vi "test_generic.vi"() -> (0 "error out":errorcluster)   [LabVIEW 2010, in "GenericInstrument.lvclass"]
uses:
  GenericInstrument.lvclass
  main/labview_source/type_definitions/clusters/controls_refs.ctl
  common/classes/ErrorController/ErrorController/ErrorController.lvclass
  common/classes/GenericToplevelComponent/GenericToplevelComponent/common_trigger_enum.ctl
  common/classes/XMLElement/XMLElement/XMLElement.lvclass
  common/classes/ErrorController/ErrorController/class_data.vi
  common/classes/GenericComponent/GenericComponent/GenericComponent.lvclass
  common/classes/GenericToplevelComponent/GenericToplevelComponent/GenericToplevelComponent.lvclass
panel:
  out "error loaded?":bool
  in  "create OME XML button":bool
  out "OME XML":string
  in  "scan start button":bool
  in  "create button":bool
  in  "stop button":bool
  # "Test Instrument"
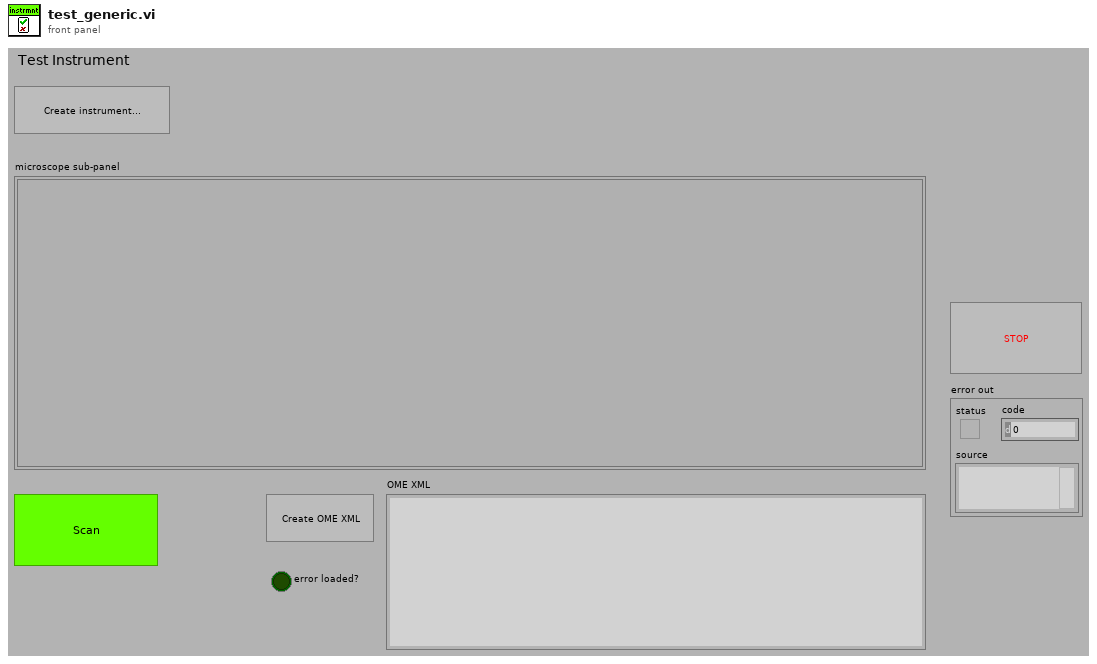
[diagram p1: front panel]
types:
  T1 = typedef "controls_refs.ctl" = cluster{"scan start button":refnum<vi>, "tabs":cluster{"main":refnum<vi>, "settings":refnum<vi>}, "subpanels":cluster{"imagingMode":refnum<vi>, "scanHead":refnum<vi>, "display":refnum<vi>, "experimentController":refnum<vi>, "instrument":refnum<vi>, "stage":refnum<vi>, "stimulator":refnum<vi>, "dataCollection":refnum<vi>, "analyser":refnum<vi>, "daq":refnum<vi>, "imageAssembler":refnum<vi>}, "drop-downs":cluster{"run mode":refnum<vi>, "imagingMode":refnum<vi>, "experimentalController":refnum<vi>, "objective":refnum<vi>}, "status lights":cluster{"experimentController":refnum<vi>, "imagingMode":refnum<vi>, "scanHead":refnum<vi>, "daq":refnum<vi>, "imageAssembler":refnum<vi>, "dataCollection":refnum<vi>, "display":refnum<vi>, "analyser":refnum<vi>, "stage":refnum<vi>, "stimulator":refnum<vi>, "instrument":refnum<vi>}, "message":refnum<vi>, "stimulator enabled?":refnum<vi>, "saving":cluster{"data folder path":refnum<vi>, "file base name":refnum<vi>, "notebook":refnum<vi>}, "progress bar":refnum<vi>, "update icon":refnum<vi>, "title":refnum<vi>, "main vi":refnum<vi>, "user":refnum<vi>, "exit_button":refnum<vi>, "CPU usage %":refnum<vi>}
  T2 = typedef "GenericToplevelComponent.lvclass/common_trigger_enum.ctl" = enum16{"NULL", "initialise", "terminate", "fetch command", "fetch data", "attach observer", "register as observer", "detach observer", "acknowledge", "start", "stop", "sweep started", "sweep finished", "experiment started", "experiment stopped"}
  T3 = typedef "XComponentSpecification.xctl/data.ctl" = cluster{"class path":string, "configuration":string, "label":string, "settings name":string}
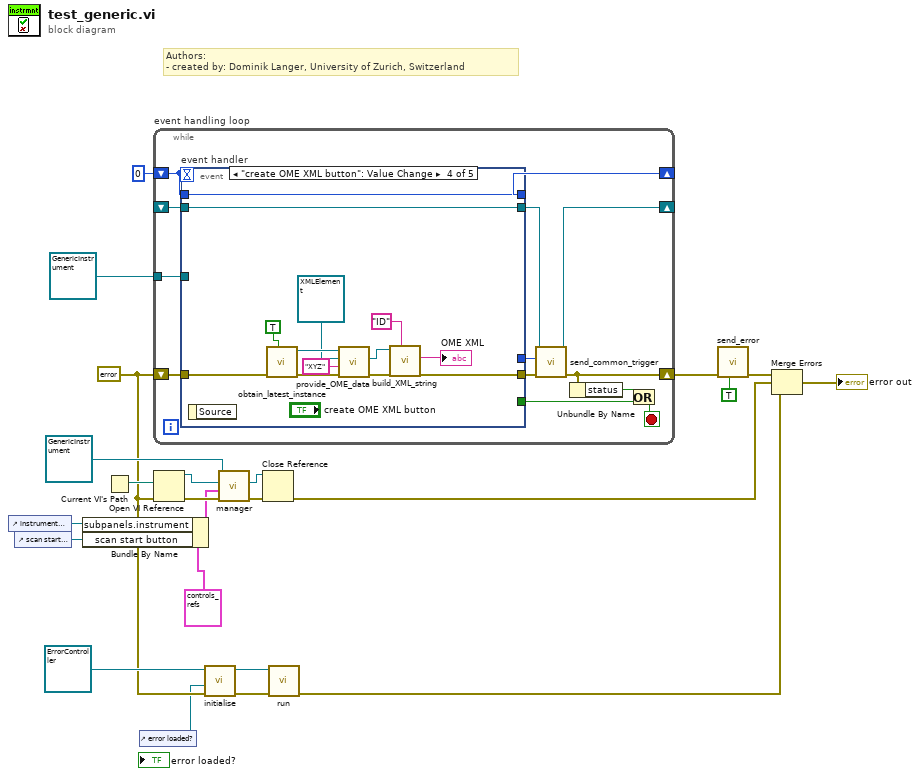
[diagram p0: block diagram]
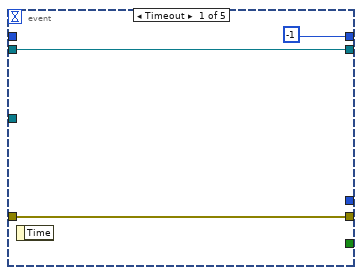
[diagram p2: hidden frame]
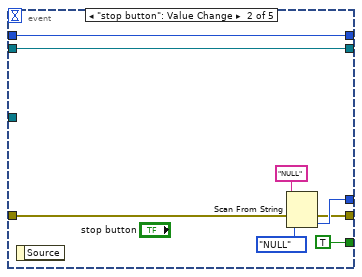
[diagram p3: hidden frame]
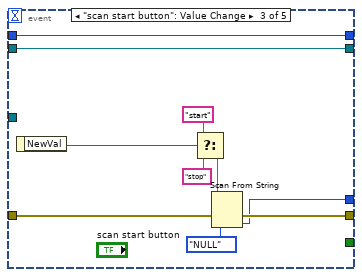
[diagram p4: hidden frame]
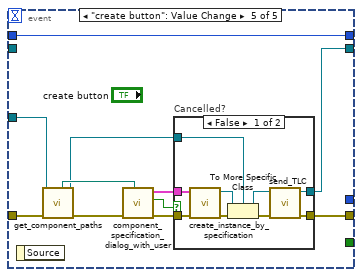
[diagram p5: hidden frame]
diagram:
  w3 = errorcluster {"status"=FALSE, "code"=0, "source"=""} ("error out")
  # "Authors: \n- created by: Dominik Langer, University of Zurich, Switzerland"
  n1 = control-ref of="instrument sub-panel"() -> (w21:refnum<vi>)
  n2 = control-ref of="scan start button"() -> (w19:refnum<vi>)
  n3 = Bundle By Name(cluster=T1 {"scan start button"=refnum, "tabs"={"main"=refnum, "settings"=refnum}, "subpanels"={"imagingMode"=refnum, "scanHead"=refnum, "display"=refnum, "experimentController"=refnum, "instrument"=refnum, "stage"=refnum, "stimulator"=refnum, "dataCollection"=refnum, "analyser"=refnum, "daq"=refnum, "imageAssembler"=refnum}, "drop-downs"={"run mode"=refnum, "imagingMode"=refnum, "experimentalController"=refnum, "objective"=refnum}, "status lights"={"experimentController"=refnum, "imagingMode"=refnum, "scanHead"=refnum, "daq"=refnum, "imageAssembler"=refnum, "dataCollection"=refnum, "display"=refnum, "analyser"=refnum, "stage"=refnum, "stimulator"=refnum, "instrument"=refnum}, "message"=refnum, "stimulator enabled?"=refnum, "saving"={"data folder path"=refnum, "file base name"=refnum, "notebook"=refnum}, "progress bar"=refnum, "update icon"=refnum, "title"=refnum, "main vi"=refnum, "user"=refnum, "exit_button"=refnum, "CPU usage %"=refnum} ("control references"), "subpanels.instrument"=w21, "scan start button"=w19) -> (w14:T1)
  n4 = Current VI's Path() -> (path=w16:path)
  n5 = control-ref of="error loaded?"() -> (w2:refnum<vi>)
  n6 = while "event handling loop" {
    shift-right: [w27] -> w6
    shift-left: w3 -> [w36]
    shift-right: [w34] -> _
    shift-left: 0 -> [w35]
    shift-right: [w30] -> _
    shift-left: _ -> [w33]
    tunnel: refnum<class "GenericInstrument.lvclass"> refnum ("GenericInstrument.lvclass") -> [w28]
    stop <- w25 stop-if-true
    n7 = event "event handler" shown="[3] \"create OME XML button\": Value Change" {
      selector: _ -> [_ _ _ _ _]
      dyn-events: _ -> [_ _ _ _ _]
      timeout: w35 -> [_ _ _ _ _]
      tunnel: w36 -> [w37 w41 w53 w68 w75]
      tunnel: [-1 w47 w57 w70 w81] -> w34
      tunnel: w35 -> [_ w47 w57 w70 w81]
      tunnel: [w37 w40 w52 w61 w80] -> w31
      tunnel: [_ TRUE _ _ _] -> w24
      tunnel: w33 -> [w38 w45 w55 w69 _]
      tunnel: [w38 w45 w55 w69 w79] -> w32
      tunnel: [_ w42 w48 _ _] -> w29
      tunnel: w28 -> [_ _ _ _ w74]
      event Timeout {
        n8 = event-data() -> ()  [unwired: 2 out]
      }
      event "stop button": Value Change {
        n9 = event-data() -> ()  [unwired: 2 out]
        n10 = Scan From String(input string="NULL", error in=w41, default 1=common_trigger_enum."NULL" ("f")) -> (error out=w40:errorcluster, output 1=w42:T2)  [unwired: 2 in, 2 out]
      }
      event "scan start button": Value Change {
        n11 = event-data() -> ("NewVal"=w56:bool)  [unwired: 1 out]
        n12 = Select(t="start", s=w56, f="stop") -> (s? t:f=w51:string)
        n13 = Scan From String(input string=w51, error in=w53, default 1=common_trigger_enum."NULL" ("f")) -> (error out=w52:errorcluster, output 1=w48:T2)  [unwired: 2 in, 2 out]
      }
      event "create OME XML button": Value Change {
        n14 = event-data() -> ()  [unwired: 2 out]
        n15 = call "obtain_latest_instance.vi"("quick, but maybe outdated?"=TRUE, "error in (no error)"=w68) -> ("error out"=w66:errorcluster, "microscope"=w65:refnum<class "GenericInstrument.lvclass">)  [unwired: 8 in]
        n16 = call-dynamic "provide_OME_data.vi"("error in (no error)"=w66, "structuredAttribute string in"="XYZ" ("image ID"), "OME element in"=refnum<class "XMLElement.lvclass"> refnum ("XMLElement.lvclass"), "GenericPlugin in"=w65) -> ("error out"=w62:errorcluster, "OME element out"=w60:refnum<class "XMLElement.lvclass">)  [unwired: 4 in, 2 out]
        n17 = call "build_XML_string.vi"("ID tag"="ID" ("id parameter name"), "error in (no error)"=w62, "Element in"=w60) -> ("error out"=w61:errorcluster, "string"=→"OME XML":string)  [unwired: 6 in, 1 out]
      }
      event "create button": Value Change {
        n18 = event-data() -> ()  [unwired: 2 out]
        n19 = call-dynamic "get_component_paths.vi"("error in (no error)"=w75, "GenericComponent in"=w74) -> ("error out"=w77:errorcluster, "GenericComponent out"=w73:refnum<class "GenericInstrument.lvclass">, "component type directory"=w78:path)  [unwired: 4 in, 3 out]
        n20 = call "component_specification_dialog_with_user.vi"("start path"=w78, "error in (no error)"=w77) -> ("error out"=w76:errorcluster, "cancelled?"=w71:bool, "component specification out"=w72:T3)  [unwired: 7 in]
        n21 = case "Cancelled?" shown="False" w71 {
          tunnel: [w88 w92] -> w80
          tunnel: [w85 w91] -> w79
          tunnel: w76 -> [w84 w92]
          tunnel: w73 -> [w83 w91]
          tunnel: w72 -> [w82 _]
          frame False {
            n22 = call "create_instance_by_specification.vi"("error in (no error)"=w84, "component specification"=w82) -> ("error out"=w90:errorcluster, "GenericPlugin out"=w87:refnum<class "GenericComponent.lvclass">)  [unwired: 7 in, 1 out]
            n23 = To More Specific Class(target class=w83, reference=w87, error in=w90) -> (specific class reference=w86:refnum<class "GenericInstrument.lvclass">, error out=w89:errorcluster)
            n24 = call-dynamic "send_TLC.vi"("error in (no error)"=w89, "GenericToplevelComponent in"=w86) -> ("error out"=w88:errorcluster, "GenericToplevelComponent out"=w85:refnum<class "GenericInstrument.lvclass">)  [unwired: 8 in]
          }
          frame True {
          }
        }
      }
    }
    n25 = call-dynamic "send_common_trigger.vi"("error in (no error)"=w31, "trigger"=w29, "GenericToplevelComponent in"=w32) -> ("error out"=w27:errorcluster, "GenericToplevelComponent out"=w30:refnum<class "GenericInstrument.lvclass">)  [unwired: 6 in, 1 out]
    n26 = Unbundle By Name(w27) -> ("status"=w26:bool)
    n27 = Or(x=w26, y=w24) -> (x .or. y?=w25:bool)
  }
  n28 = Open VI Reference(vi path=w16, error in (no error)=w3) -> (vi reference=w13:refnum<vi>, error out=w15:errorcluster)  [unwired: 4 in]
  n29 = call-dynamic "initialise.vi"("error in (no error)"=w3, "error boolean"=w2, "ErrorController in"=refnum<class "ErrorController.lvclass"> refnum) -> ("error out"=w8:errorcluster, "ErrorController out"=w7:refnum<class "ErrorController.lvclass">)  [unwired: 7 in]
  n30 = call-dynamic "manager.vi"("error in (no error)"=w15, "control references"=w14, "top-level VI ref in"=w13, "GenericToplevelComponent in"=refnum<class "GenericInstrument.lvclass"> refnum ("GenericInstrument.lvclass")) -> ("error out"=w12:errorcluster, "top-level VI ref out"=w11:refnum<vi>)  [unwired: 5 in, 1 out]
  n31 = Close Reference(reference=w11, error in (no error)=w12) -> (error out=w17:errorcluster)
  n32 = call "run.vi"("error in (no error)"=w8, "ErrorController in"=w7) -> ("error out"=w1:errorcluster)  [unwired: 8 in, 1 out]
  n33 = call "send_error.vi"("last error? (F)"=TRUE, "error in (no error)"=w6) -> ("error out"=w5:errorcluster)  [unwired: 9 in]
  n34 = Merge Errors(w5, w17, w1) -> (→"error out":errorcluster)
